vi "Main_flow_full.vi"() -> ()   [LabVIEW 2022 SP3]
uses:
  <vilib>/DAQmx/create/channels.llb/DAQmx Create Channel (DI-Digital Input).vi
  <vilib>/DAQmx/read.llb/DAQmx Read (Digital Bool 1Line 1Point).vi
  <vilib>/DAQmx/write.llb/DAQmx Write (Digital Bool 1Line 1Point).vi
  <vilib>/DAQmx/create/channels.llb/DAQmx Create Channel (DO-Digital Output).vi
panel:
  in  "UP DOWN 2":tag
  in  "UP DOWN 1":tag
  in  "Buzzer":tag
  out "Counter":dbl
  out "OUT COUNT":dbl
  out "IN COUNT":dbl
  in  "Door IR 2":tag
  in  "Door IR 1":tag
  in  "temp":dbl
  in  "Trigger Period(sec)":dbl
  out "Current Time":dbl
  in  "Mode":dbl
  in  "stop":bool
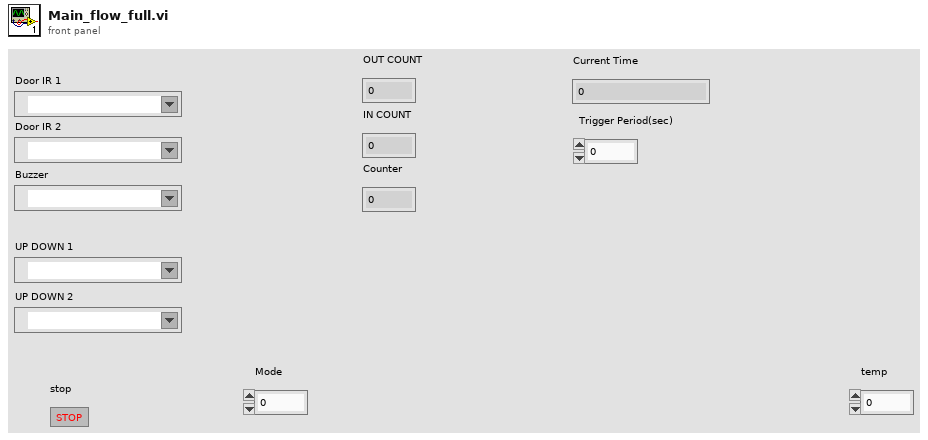
[diagram p1: front panel]
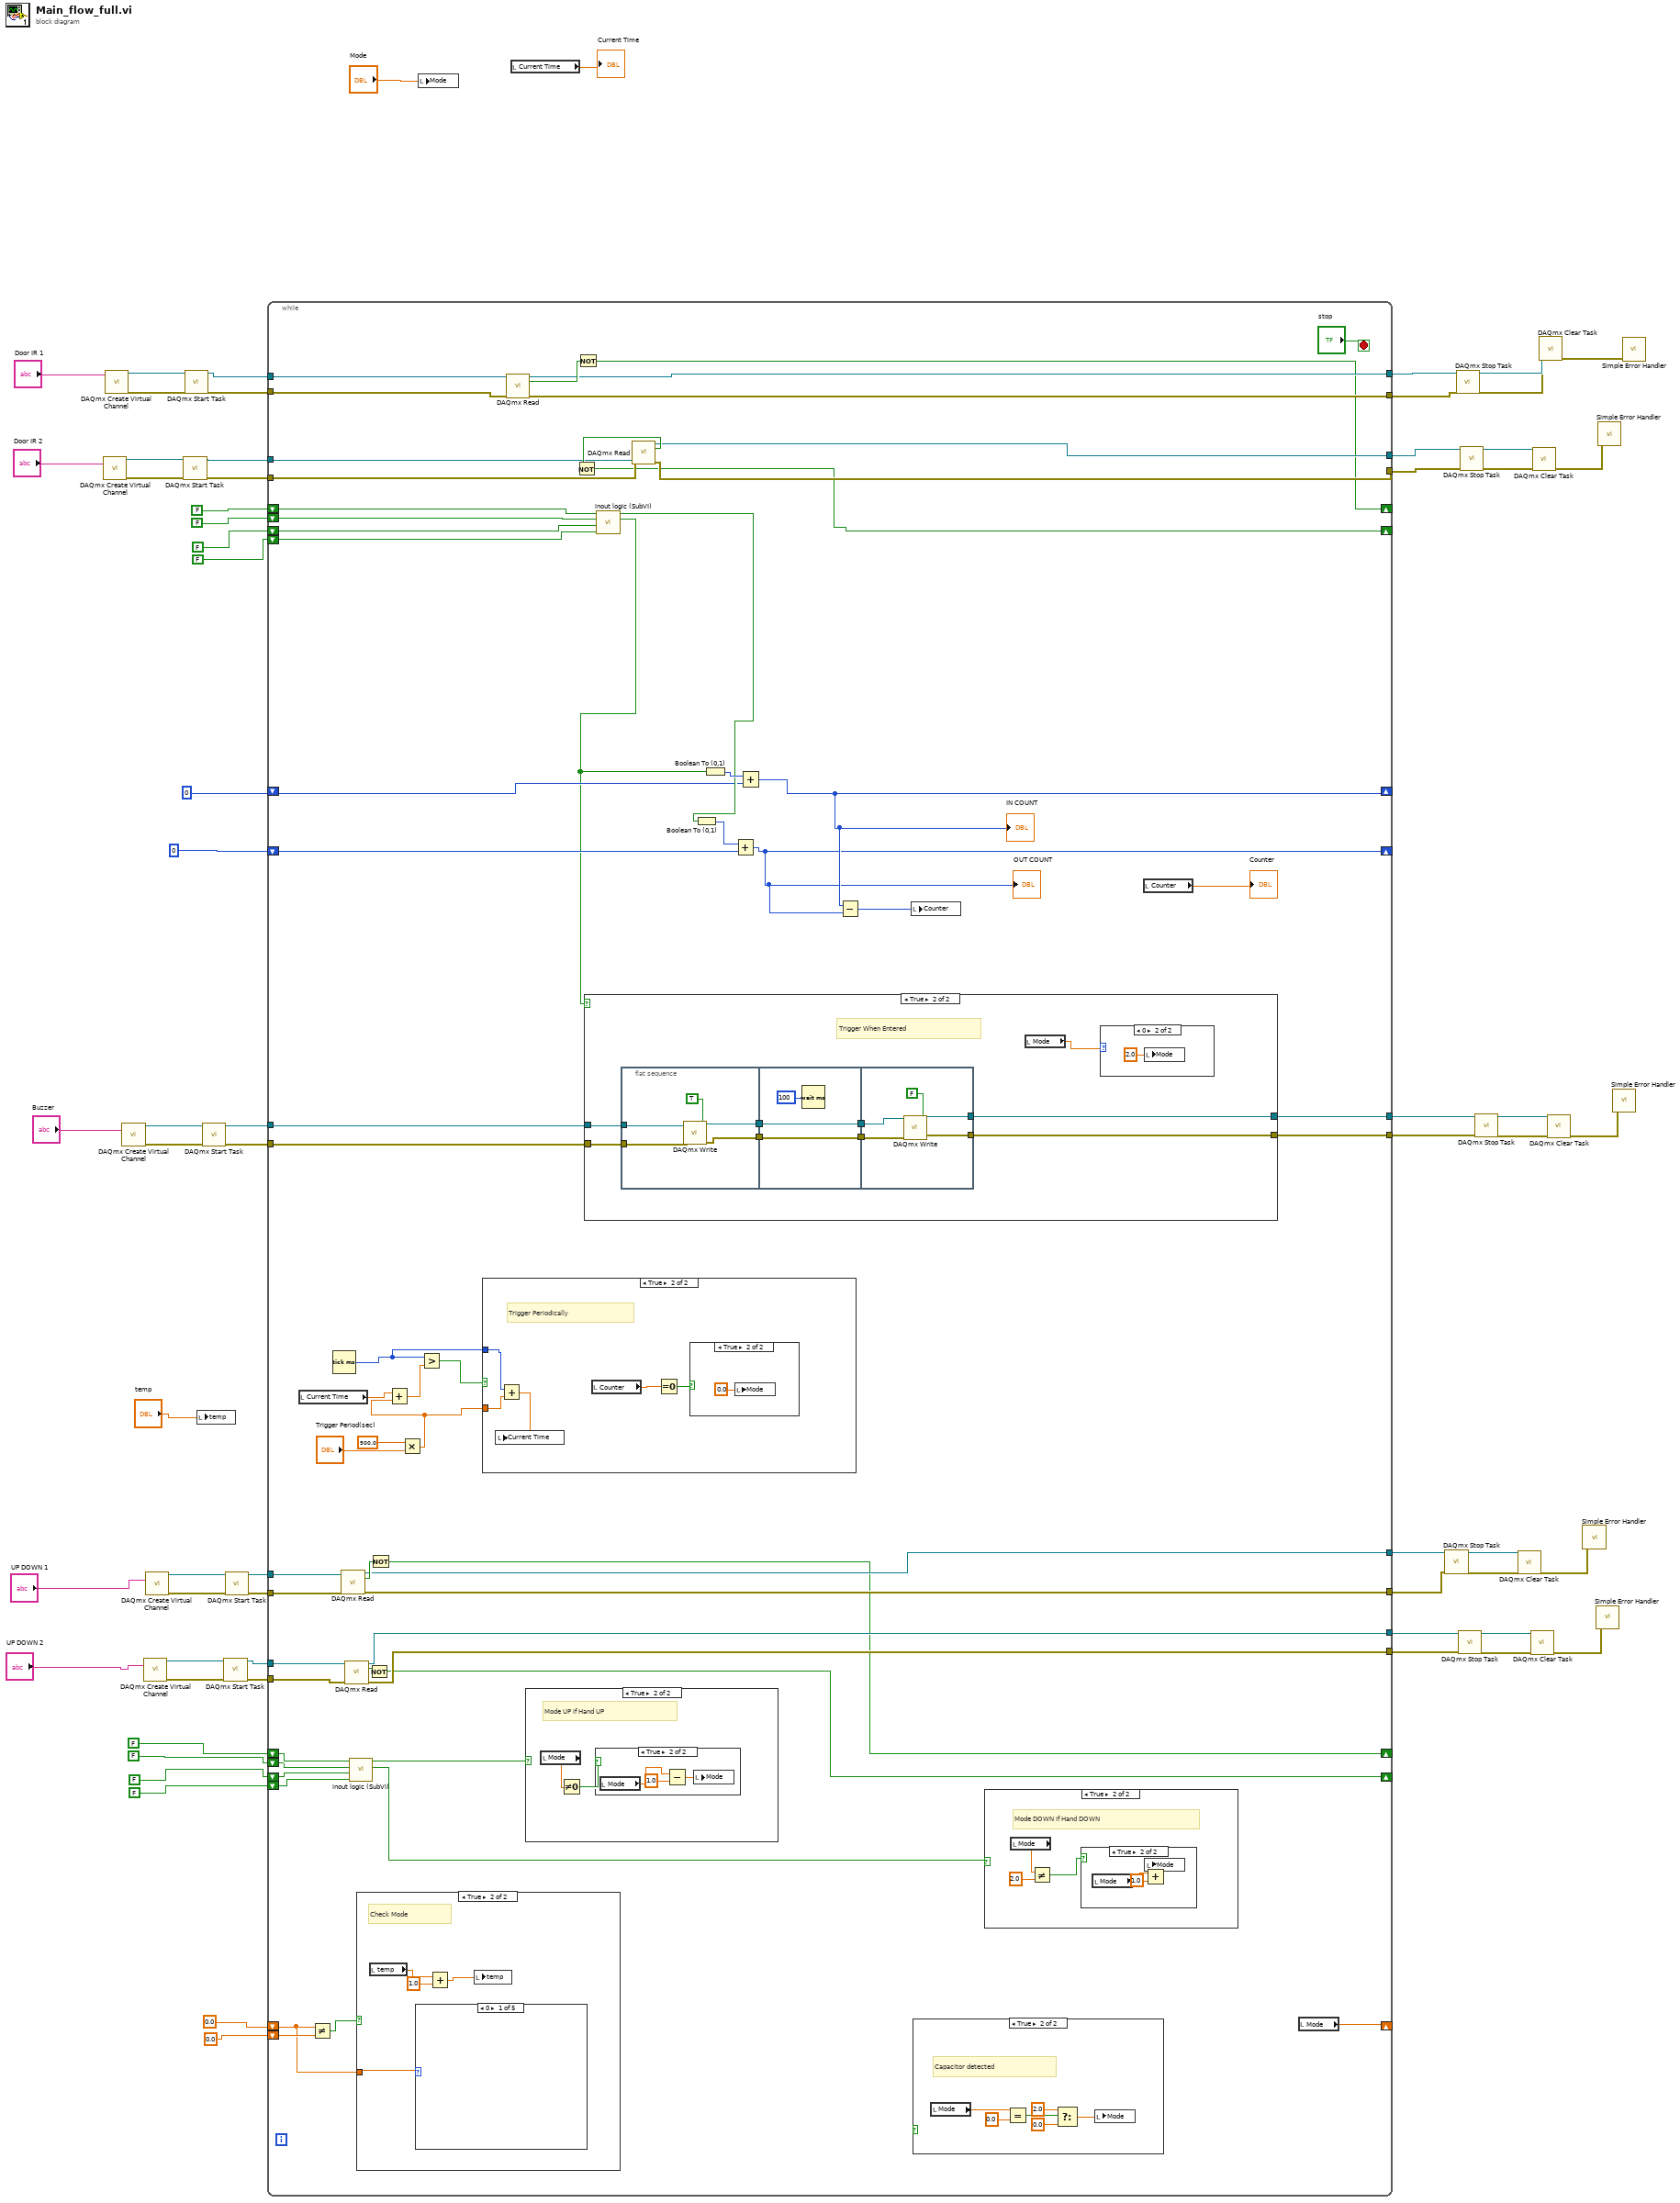
[diagram p0: block diagram]
diagram:
  n1 = call-poly <vilib>:"DAQmx Create Virtual Channel.vi"("lines"="Door IR 2") -> ("task out"=w58:refnum<k21>, "error out"=w52:errorcluster)  [unwired: 13 in]
  n2 = call-poly <vilib>:"DAQmx Create Virtual Channel.vi"("lines"="Door IR 1") -> ("task out"=w60:refnum<k21>, "error out"=w54:errorcluster)  [unwired: 13 in]
  n3 = call-poly <vilib>:"DAQmx Create Virtual Channel.vi"("lines"="Buzzer") -> ("task out"=w35:refnum<k21>, "error out"=w33:errorcluster)  [unwired: 13 in]
  n4 = call-poly <vilib>:"DAQmx Create Virtual Channel.vi"("lines"="UP DOWN 2") -> ("task out"=w24:refnum<k21>, "error out"=w22:errorcluster)  [unwired: 13 in]
  n5 = call-poly <vilib>:"DAQmx Create Virtual Channel.vi"("lines"="UP DOWN 1") -> ("task out"=w25:refnum<k21>, "error out"=w23:errorcluster)  [unwired: 13 in]
  n6 = call <vilib>:"DAQmx Start Task.vi"("task/channels in"=w58, "error in"=w52) -> ("task out"=w55:refnum<k21>, "error out"=w51:errorcluster)  [unwired: 12 in]
  n7 = call <vilib>:"DAQmx Start Task.vi"("task/channels in"=w60, "error in"=w54) -> ("task out"=w56:refnum<k21>, "error out"=w53:errorcluster)  [unwired: 12 in]
  n8 = local write "temp"("temp") -> ()
  n9 = call <vilib>:"DAQmx Start Task.vi"("task/channels in"=w35, "error in"=w33) -> ("task out"=w32:refnum<k21>, "error out"=w31:errorcluster)  [unwired: 12 in]
  n10 = call <vilib>:"DAQmx Start Task.vi"("task/channels in"=w24, "error in"=w22) -> ("task out"=w17:refnum<k21>, "error out"=w16:errorcluster)  [unwired: 12 in]
  n11 = call <vilib>:"DAQmx Start Task.vi"("task/channels in"=w25, "error in"=w23) -> ("task out"=w19:refnum<k21>, "error out"=w18:errorcluster)  [unwired: 12 in]
  n12 = while {
    shift-right: [w117] -> _
    shift-left: 0.0 ("Mode") -> [w114]
    shift-left: 0.0 ("Mode") -> [w116]
    tunnel: w56 -> [w108]
    tunnel: w55 -> [w107]
    tunnel: w53 -> [w106]
    tunnel: w51 -> [w105]
    tunnel: [w104] -> w50
    tunnel: [w103] -> w49
    tunnel: [w102] -> w45
    tunnel: [w101] -> w41
    shift-right: [w92] -> _
    shift-left: FALSE -> [w100]
    shift-left: FALSE -> [w99]
    shift-right: [w95] -> _
    shift-left: FALSE -> [w98]
    shift-left: FALSE -> [w68]
    shift-right: [w94] -> _
    shift-left: 0 -> [w97]
    shift-right: [w93] -> _
    shift-left: 0 -> [w96]
    tunnel: w32 -> [w88]
    tunnel: w31 -> [w87]
    tunnel: [w86] -> w27
    tunnel: [w85] -> w26
    shift-right: [w74] -> _
    shift-left: FALSE -> [w72]
    shift-right: [w73] -> _
    shift-left: FALSE -> [w70]
    shift-left: FALSE -> [w71]
    shift-left: FALSE -> [w69]
    tunnel: w19 -> [w82]
    tunnel: w18 -> [w81]
    tunnel: w17 -> [w80]
    tunnel: w16 -> [w79]
    tunnel: [w78] -> w9
    tunnel: [w77] -> w8
    tunnel: [w76] -> w7
    tunnel: [w75] -> w6
    stop <- "stop" stop-if-true
    n13 = local read "Current Time"() -> (w124:dbl)
    n14 = Not Equal?(x=w114, y=w116) -> (x != y?=w115:bool)
    n15 = Tick Count (ms)() -> (millisecond timer value=w122:u32)
    n16 = call-poly <vilib>:"DAQmx Read.vi"("task/channels in"=w82, "error in"=w81) -> ("task out"=w78:refnum<k21>, "data"=w84:bool, "error out"=w77:errorcluster)  [unwired: 11 in]
    n17 = call-poly <vilib>:"DAQmx Read.vi"("task/channels in"=w80, "error in"=w79) -> ("task out"=w76:refnum<k21>, "data"=w83:bool, "error out"=w75:errorcluster)  [unwired: 11 in]
    n18 = call "inout logic (SubVI).vi"("Sensor 2 (T-2)"=w69, "Sensor 2 (T-1)"=w70, "Sensor 1 (T-2)"=w71, "Sensor 1 (T-1)"=w72) -> ("IN"=w67:bool, "OUT"=w66:bool)  [unwired: 6 in]
    n19 = case shown="True" w115 {
      tunnel: w114 -> [_ w126]
      frame False {
      }
      frame True {
        # "Check Mode"
        n20 = local read "temp"() -> (w129:dbl)
        n21 = case shown="0" w126 {
          frame 0 {
          }
          frame 1 {
          }
          frame 2 {
          }
          frame 3 {
          }
          frame Default {
          }
        }
        n22 = Add(x=w129, y=1.0) -> (x+y=w128:dbl)
        n23 = local write "temp"(w128) -> ()
      }
    }
    n24 = Not(x=w83) -> (.not. x?=w73:bool)
    n25 = Not(x=w84) -> (.not. x?=w74:bool)
    n26 = Multiply(x=500.0, y="Trigger Period(sec)") -> (x*y=w118:dbl)
    n27 = Add(x=w124, y=w118) -> (x+y=w121:dbl)
    n28 = Greater?(x=w122, y=w121) -> (0:w123:bool)
    n29 = case shown="True" w123 {
      tunnel: w122 -> [_ w144]
      tunnel: w118 -> [_ w143]
      frame False {
      }
      frame True {
        # "Trigger Periodically"
        n30 = Add(x=w144, y=w143) -> (x+y=w145:dbl)
        n31 = local write "Current Time"(w145) -> ()
        n32 = local read "Counter"() -> (w142:dbl)
        n33 = Equal To 0?(x=w142) -> (x = 0?=w141:bool)
        n34 = case shown="True" w141 {
          frame False {
          }
          frame True {
            n35 = local write "Mode"(0.0 ("Mode")) -> ()
          }
        }
      }
    }
    n36 = call-poly <vilib>:"DAQmx Read.vi"("task/channels in"=w108, "error in"=w106) -> ("task out"=w104:refnum<k21>, "data"=w113:bool, "error out"=w103:errorcluster)  [unwired: 11 in]
    n37 = case shown="True" w66 {
      frame False {
      }
      frame True {
        # "Mode UP if Hand UP"
        n38 = local read "Mode"() -> (w131:dbl)
        n39 = Not Equal To 0?(x=w131) -> (x != 0?=w130:bool)
        n40 = case shown="True" w130 {
          frame False {
          }
          frame True {
            n41 = local read "Mode"() -> (w133:dbl)
            n42 = Subtract(x=w133, y=1.0) -> (x-y=w132:dbl)
            n43 = local write "Mode"(w132) -> ()
          }
        }
      }
    }
    n44 = Not(x=w113) -> (.not. x?=w92:bool)
    n45 = call "inout logic (SubVI).vi"("Sensor 2 (T-2)"=w68, "Sensor 2 (T-1)"=w98, "Sensor 1 (T-2)"=w99, "Sensor 1 (T-1)"=w100) -> ("IN"=w89:bool, "OUT"=w109:bool)  [unwired: 6 in]
    n46 = case shown="True" w89 {
      tunnel: w88 -> [_ w155]
      tunnel: w87 -> [_ w154]
      tunnel: [_ w149] -> w86
      tunnel: [_ w148] -> w85
      frame False {
      }
      frame True {
        # "Trigger When Entered"
        n47 = flat-sequence {
          tunnel: w155 -> [w160]
          tunnel: w154 -> [w159]
          tunnel: [w158] -> w152
          tunnel: [w157] -> w150
          tunnel: [w163] -> w153
          tunnel: w152 -> [w163]
          tunnel: [w162] -> w151
          tunnel: w150 -> [w162]
          tunnel: w153 -> [w168]
          tunnel: w151 -> [w167]
          tunnel: [w166] -> w149
          tunnel: [w165] -> w148
          frame #0 {
            n48 = call-poly <vilib>:"DAQmx Write.vi"("task/channels in"=w160, "data"=TRUE, "error in"=w159) -> ("task out"=w158:refnum<k21>, "error out"=w157:errorcluster)  [unwired: 10 in, 1 out]
          }
          frame #1 {
            n49 = Wait (ms)(milliseconds to wait=u32 100) -> ()  [unwired: 1 out]
          }
          frame #2 {
            n50 = call-poly <vilib>:"DAQmx Write.vi"("task/channels in"=w168, "data"=FALSE, "error in"=w167) -> ("task out"=w166:refnum<k21>, "error out"=w165:errorcluster)  [unwired: 10 in, 1 out]
          }
        }
        n51 = local read "Mode"() -> (w147:dbl)
        n52 = case shown="0" w147 {
          frame Default {
          }
          frame 0 {
            n53 = local write "Mode"(2.0 ("Mode")) -> ()
          }
        }
      }
    }
    n54 = call-poly <vilib>:"DAQmx Read.vi"("task/channels in"=w107, "error in"=w105) -> ("task out"=w102:refnum<k21>, "data"=w112:bool, "error out"=w101:errorcluster)  [unwired: 11 in]
    n55 = Not(x=w112) -> (.not. x?=w95:bool)
    n56 = Boolean To (0,1)(Boolean=w109) -> (0, 1=w110:i16)
    n57 = Boolean To (0,1)(Boolean=w89) -> (0, 1=w111:i16)
    n58 = Add(x=w110, y=w96) -> (x+y=w93:i32)
    "OUT COUNT" <- w93
    n59 = Add(x=w111, y=w97) -> (x+y=w94:i32)
    "IN COUNT" <- w94
    n60 = Subtract(x=w94, y=w93) -> (x-y=w91:i32)
    n61 = local write "Counter"(w91) -> ()
    n62 = case shown="True" {
      selector: _ -> [_ _]
      frame False {
      }
      frame True {
        # "Capacitor detected"
        n63 = local read "Mode"() -> (w175:dbl)
        n64 = Equal?(x=w175, y=0.0) -> (x = y?=w173:bool)
        n65 = Select(t=2.0, s=w173, f=0.0) -> (s? t:f=w172:dbl)
        n66 = local write "Mode"(w172) -> ()
      }
    }
    n67 = case shown="True" w67 {
      frame False {
      }
      frame True {
        # "Mode DOWN if Hand DOWN"
        n68 = local read "Mode"() -> (w137:dbl)
        n69 = Not Equal?(x=w137, y=2.0) -> (x != y?=w135:bool)
        n70 = case shown="True" w135 {
          frame False {
          }
          frame True {
            n71 = local read "Mode"() -> (w140:dbl)
            n72 = Add(x=w140, y=1.0) -> (x+y=w138:dbl)
            n73 = local write "Mode"(w138) -> ()
          }
        }
      }
    }
    n74 = local read "Counter"() -> (→"Counter":dbl)
    n75 = local read "Mode"() -> (w117:dbl)
  }
  n76 = local write "Mode"("Mode") -> ()
  n77 = local read "Current Time"() -> (→"Current Time":dbl)
  n78 = call <vilib>:"DAQmx Stop Task.vi"("task/channels in"=w9, "error in"=w8) -> ("task out"=w15:refnum<k21>, "error out"=w13:errorcluster)  [unwired: 12 in]
  n79 = call <vilib>:"DAQmx Stop Task.vi"("task/channels in"=w50, "error in"=w49) -> ("task out"=w48:refnum<k21>, "error out"=w47:errorcluster)  [unwired: 12 in]
  n80 = call <vilib>:"DAQmx Stop Task.vi"("task/channels in"=w7, "error in"=w6) -> ("task out"=w12:refnum<k21>, "error out"=w10:errorcluster)  [unwired: 12 in]
  n81 = call <vilib>:"DAQmx Stop Task.vi"("task/channels in"=w45, "error in"=w41) -> ("task out"=w44:refnum<k21>, "error out"=w42:errorcluster)  [unwired: 12 in]
  n82 = call <vilib>:"DAQmx Stop Task.vi"("task/channels in"=w27, "error in"=w26) -> ("task out"=w30:refnum<k21>, "error out"=w28:errorcluster)  [unwired: 12 in]
  n83 = call <vilib>:"DAQmx Clear Task.vi"("task in"=w15, "error in"=w13) -> ("error out"=w14:errorcluster)  [unwired: 13 in]
  n84 = call <vilib>:"DAQmx Clear Task.vi"("task in"=w12, "error in"=w10) -> ("error out"=w11:errorcluster)  [unwired: 13 in]
  n85 = call <vilib>:"DAQmx Clear Task.vi"("task in"=w44, "error in"=w42) -> ("error out"=w43:errorcluster)  [unwired: 13 in]
  n86 = call <vilib>:"DAQmx Clear Task.vi"("task in"=w48, "error in"=w47) -> ("error out"=w46:errorcluster)  [unwired: 13 in]
  n87 = call <vilib>:"DAQmx Clear Task.vi"("task in"=w30, "error in"=w28) -> ("error out"=w29:errorcluster)  [unwired: 13 in]
  n88 = call <vilib>:"Simple Error Handler.vi"("error in (no error)"=w14) -> ()  [unwired: 4 in, 5 out]
  n89 = call <vilib>:"Simple Error Handler.vi"("error in (no error)"=w11) -> ()  [unwired: 4 in, 5 out]
  n90 = call <vilib>:"Simple Error Handler.vi"("error in (no error)"=w43) -> ()  [unwired: 4 in, 5 out]
  n91 = call <vilib>:"Simple Error Handler.vi"("error in (no error)"=w29) -> ()  [unwired: 4 in, 5 out]
  n92 = call <vilib>:"Simple Error Handler.vi"("error in (no error)"=w46) -> ()  [unwired: 4 in, 5 out]
